vi "Servo.vi"() -> ()   [LabVIEW 2009]
uses:
  <vilib>/eio/EIONode/EIONode.xnode
  <vilib>/rvi/eio/nirviEIOImplementation/nirviEIOImplementation.xnode
  <vilib>/rvi/eio/common/nirviEmuTemplateMethod_noerrors.vi
  <vilib>/rvi/eio/common/nirviEmuClasses.ctl
panel:
  in  "servo 6":u32=1500
  in  "Count(uSec)":u32=5000
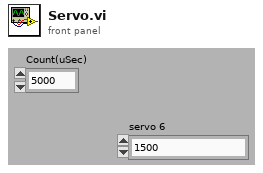
[diagram p1: front panel]
types:
  T1 = typedef "nirviEmuClasses.ctl" = enum16{"IO Read", "IO Write", "Method", "Property Read", "Property Write"}
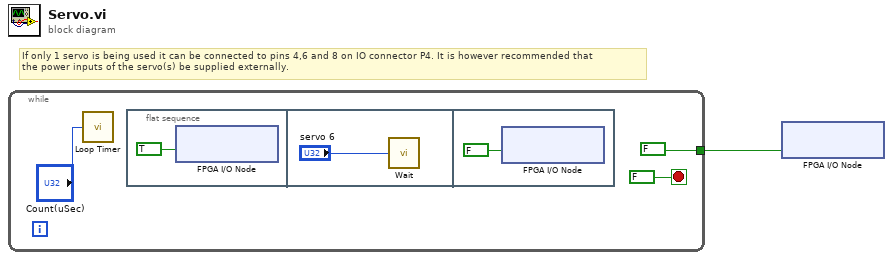
[diagram p0: block diagram]
diagram:
  # "If only 1 servo is being used it can be connected to pins 4,6 and 8 on IO connector P4. It is however recommended that\nthe power inputs of the servo(s) be supplied externally."
  n1 = while {
    tunnel: [FALSE ("Mod1/DO0")] -> w1
    stop <- FALSE stop-if-true
    n2 = call "Loop Timer"("Count(uSec)"="Count(uSec)") -> ()  [unwired: 1 out]
    n3 = flat-sequence {
      frame #0 {
        n4 = xnode "FPGA I/O Node"("Mod1/DO0"=TRUE) -> ()  [unwired: 1 in, 1 out]
      }
      frame #1 {
        n5 = call "Wait"("Count(uSec)"="servo 6") -> ()  [unwired: 1 out]
      }
      frame #2 {
        n6 = xnode "FPGA I/O Node"("Mod1/DO0"=FALSE) -> ()  [unwired: 1 in, 1 out]
      }
    }
  }
  n7 = xnode "FPGA I/O Node"("Mod1/DO0"=w1) -> ()  [unwired: 1 in, 1 out]
